vi "Set Read Only.vi"(8 "Error In":errorcluster, 10 "Read Only":bool, 11 "Dual Mode Thermometer in":refnum<class "Dual Mode Thermometer.lvclass">) -> (0 "Error Out":errorcluster, 3 "Dual Mode Thermometer out":refnum<class "Dual Mode Thermometer.lvclass">)   [LabVIEW 2014, in "Dual Mode Thermometer.lvclass"]
doc: "Makes this thermometer user-editable (False) or read-only (True).\n\n\nCopyright (c) 2019 Sze Howe Koh.\nThis code is licensed under the MIT license."
uses:
  Dual Mode Thermometer.lvclass
  Dual Mode Thermometer.lvclass/Dual Mode Thermometer.ctl
  <vilib>/addons/LQ/Qt Widgets/QWidget/QWidget.lvclass
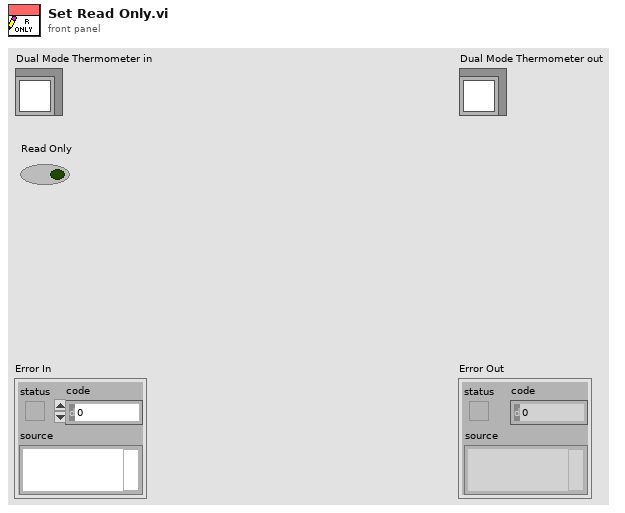
[diagram p1: front panel]
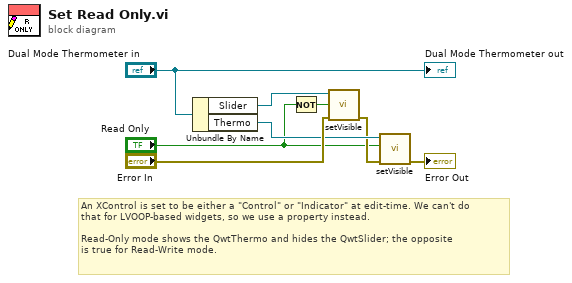
[diagram p0: block diagram]
diagram:
  # "An XControl is set to be either a \"Control\" or \"Indicator\" at edit-time. We can't do\nthat for LVOOP-based widgets, so we use a property instead.\n\nRead-Only mode shows the QwtThermo and hides the QwtSlider; the opposite\nis true for Read-Write mode."
  n1 = Unbundle By Name("Dual Mode Thermometer in") -> ("Slider"=w7:refnum<class "QwtSlider.lvclass">, "Thermo"=w5:refnum<class "QwtThermo.lvclass">)
  n2 = Not(x="Read Only") -> (.not. x?=w2:bool)
  n3 = call <vilib>:"setVisible.vi"("Error In"="Error In", "visible"=w2, "QWidget In"=w7) -> ("Error Out"=w4:errorcluster)  [unwired: 7 in, 1 out]
  n4 = call <vilib>:"setVisible.vi"("Error In"=w4, "visible"="Read Only", "QWidget In"=w5) -> ("Error Out"=→"Error Out":errorcluster)  [unwired: 7 in, 1 out]
  "Dual Mode Thermometer out" <- "Dual Mode Thermometer in"
